vi "While Loop Stop Example.vi"() -> ()   [LabVIEW 2019]
uses:
  <vilib>/gpm_packages/@cs/test-executive/Source/Test Executive/TestExecutive/Test Executive.lvclass
  C:/Program Files/National Instruments/LabVIEW 2019/vi.lib/gpm_packages/@cs/test-executive/Source/Test Executive/ITestExecutive/ITest Executive.lvclass
  <vilib>/gpm_packages/@cs/run-time-assertions/Source/Assert Equal/Assert Equal.lvclass
  C:/Program Files/National Instruments/LabVIEW 2019/vi.lib/gpm_packages/@cs/run-time-assertions/Source/Assert/Assert.lvclass
  52cc7c55-fdef-40cb-9b01-06c8b27f6ce0.vi
  a0d94dfd-d8d0-4b1a-8204-38a80b6efbaa.vi
  c6de0239-6f38-4b7c-b092-4f7ec1379bf5.vi
  5f8b3cd8-e4ad-4ca2-853e-23f3d1aa975d.vi
  <vilib>/Utility/error.llb/Error Cluster From Error Code.vi
  <vilib>/gpm_packages/@cs/test-executive/Source/Test Executive/ITestExecutive/ITest Executive.lvclass
  <vilib>/gpm_packages/@cs/test-executive/Source/Test Executive/TestExecutive Ref/TestExecutive Ref.lvclass
  <vilib>/gpm_packages/@cs/test-executive/Source/Sandbox/While Loop Stop Example/Mock Executioner/Mock Executioner.lvclass
panel:
  in  "Stop":bool
  in  "Tree":string(tree)
  out "Iteration Counter":i32
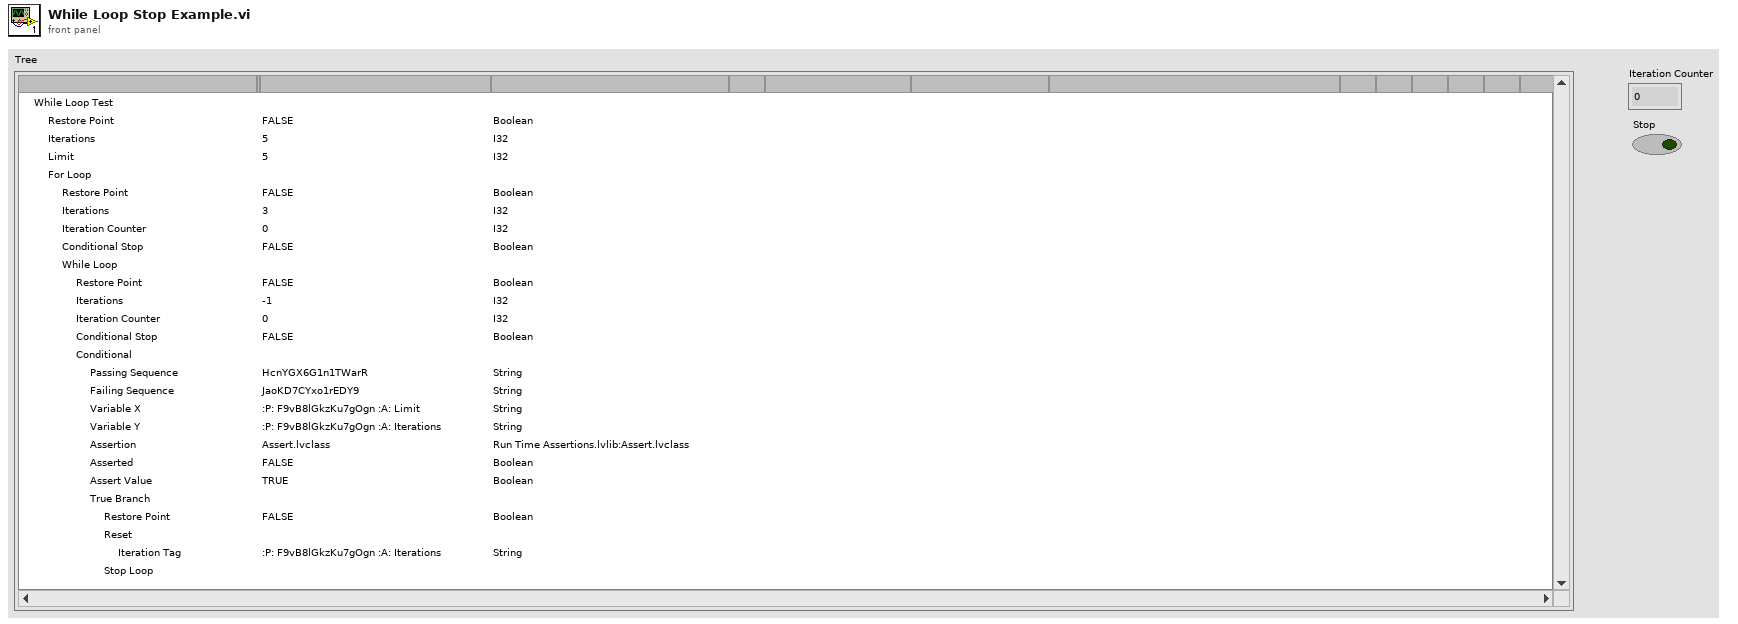
[diagram p1: front panel]
types:
  T1 = cluster{"Left Cell String":string, "Child Text":string[], "Child Tag":string, "Item Indent":i32, "Child Only?":bool, "Glyph Index":i32}[]
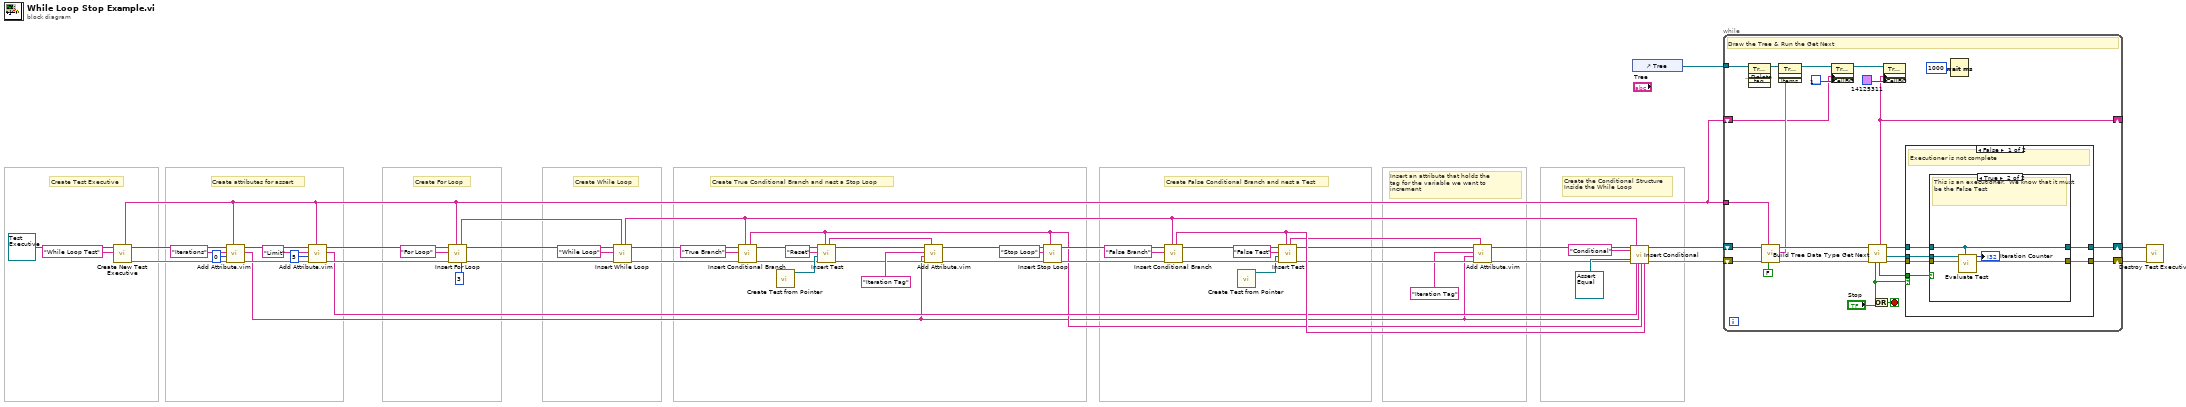
[diagram p0: block diagram]
diagram:
  # "Create For Loop"
  # "Insert an attribute that holds the\ntag for the variable we want to\nincrement"
  # "Create the Conditional Structure\nInside the While Loop"
  # "Create False Conditional Branch and nest a Test"
  # "Create True Conditional Branch and nest a Stop Loop"
  # "Create While Loop"
  # "Create attributes for assert"
  # "Create Test Executive"
  n1 = call <vilib>:"Create New Test Executive.vi"("Name"="While Loop Test", "Test Executive"=refnum<class "Test Executive.lvclass"> refnum ("Test Executive.lvlib:Test Executive.lvclass")) -> ("error out"=w54:errorcluster, "Test Executive Ref"=w55:refnum<data-value>, "Test Executive ID out"=w16:string)  [unwired: 7 in]
  n2 = call "Add Attribute.vim"("ID"=w16, "error in (no error)"=w54, "Attribute"=0, "Attribute Name"="Iterations", "Test Executive Ref"=w55) -> ("error out"=w45:errorcluster, "Attribute ID out"=w1:string, "Test Executive Ref out"=w46:refnum<data-value>)  [unwired: 3 in, 1 out]
  n3 = call "Add Attribute.vim"("ID"=w16, "error in (no error)"=w45, "Attribute"=5, "Attribute Name"="Limit", "Test Executive Ref"=w46) -> ("error out"=w22:errorcluster, "Attribute ID out"=w13:string, "Test Executive Ref out"=w20:refnum<data-value>)  [unwired: 3 in, 1 out]
  n4 = call <vilib>:"Insert For Loop.vi"("Loop Iterations"=3, "Parent ID"=w16, "error in (no error)"=w22, "Name"="For Loop", "Test Executive Ref"=w20) -> ("error out"=w21:errorcluster, "Test Executive Ref out"=w19:refnum<data-value>, "Unique ID out"=w15:string)  [unwired: 3 in, 1 out]
  n5 = call <vilib>:"Insert While Loop.vi"("Parent ID"=w15, "error in (no error)"=w21, "Name"="While Loop", "Test Executive Ref"=w19) -> ("error out"=w50:errorcluster, "Test Executive Ref out"=w51:refnum<data-value>, "Unique ID out"=w40:string)  [unwired: 4 in, 1 out]
  n6 = call <vilib>:"Insert Conditional Branch.vi"("Parent ID"=w40, "error in (no error)"=w50, "Name"="True Branch", "Test Executive Ref"=w51) -> ("error out"=w8:errorcluster, "Test Executive Ref out"=w10:refnum<data-value>, "Unique ID out"=w9:string)  [unwired: 4 in, 1 out]
  n7 = call <vilib>:"Create Test from Pointer.vi"() -> ("Test"=w12:refnum<class "Executioner.lvclass">)  [unwired: 11 in]
  n8 = call <vilib>:"Insert Test.vi"("Parent ID"=w9, "error in (no error)"=w8, "Test"=w12, "Name"="Reset", "Test Executive Ref"=w10) -> ("error out"=w4:errorcluster, "Test Executive Ref out"=w6:refnum<data-value>, "Unique ID out"=w2:string)  [unwired: 3 in, 1 out]
  n9 = call "Add Attribute.vim"("ID"=w2, "error in (no error)"=w4, "Attribute"=w1, "Attribute Name"="Iteration Tag", "Test Executive Ref"=w6) -> ("error out"=w3:errorcluster, "Test Executive Ref out"=w5:refnum<data-value>)  [unwired: 3 in, 2 out]
  n10 = call <vilib>:"Insert Stop Loop.vi"("Parent ID"=w9, "error in (no error)"=w3, "Name"="Stop Loop", "Test Executive Ref"=w5) -> ("error out"=w36:errorcluster, "Test Executive Ref out"=w14:refnum<data-value>)  [unwired: 4 in, 2 out]
  n11 = call <vilib>:"Insert Conditional Branch.vi"("Parent ID"=w40, "error in (no error)"=w36, "Name"="False Branch", "Test Executive Ref"=w14) -> ("error out"=w43:errorcluster, "Test Executive Ref out"=w42:refnum<data-value>, "Unique ID out"=w37:string)  [unwired: 4 in, 1 out]
  n12 = call <vilib>:"Create Test from Pointer.vi"() -> ("Test"=w29:refnum<class "Executioner.lvclass">)  [unwired: 11 in]
  n13 = call <vilib>:"Insert Test.vi"("Parent ID"=w37, "error in (no error)"=w43, "Test"=w29, "Name"="False Test", "Test Executive Ref"=w42) -> ("error out"=w32:errorcluster, "Test Executive Ref out"=w34:refnum<data-value>, "Unique ID out"=w30:string)  [unwired: 3 in, 1 out]
  n14 = call "Add Attribute.vim"("ID"=w30, "error in (no error)"=w32, "Attribute"=w1, "Attribute Name"="Iteration Tag", "Test Executive Ref"=w34) -> ("error out"=w31:errorcluster, "Test Executive Ref out"=w33:refnum<data-value>)  [unwired: 3 in, 2 out]
  n15 = call <vilib>:"Insert Conditional.vi"("Test Executive Ref"=w33, "Name"="Conditional", "Assertion"=refnum<class "Assert Equal.lvclass"> refnum ("Run Time Assertions.lvlib:Assert Equal.lvclass"), "error in (no error)"=w31, "Parent ID"=w40, "Variable X"=w13, "Variable Y"=w1, "Passing Executive"=w9, "Failing Executive"=w37) -> ("Test Executive Ref out"=w27:refnum<data-value>, "error out"=w26:errorcluster)  [unwired: 7 in, 2 out]
  n16 = control-ref of="Tree"() -> (w25:refnum<vi>)
  n17 = while {
    shift-right: [w78] -> w24
    shift-left: w27 -> [w76]
    shift-right: [w77] -> w23
    shift-left: w26 -> [w74]
    tunnel: w16 -> [w72]
    shift-right: [w62] -> _
    shift-left: w16 -> [w65]
    tunnel: w25 -> [w71]
    stop <- w61 stop-if-true
    # "Draw the Tree & Run the Get Next"
    n18 = invoke on="Invoke Node" class="Tree (strict)" method="Edit Tree Items.Delete"(reference=w71) -> (reference out=w70:refnum<vi>)  [unwired: 4 in, 4 out]
    n19 = call <vilib>:"Build Tree Data Type.vi"("Show IDs (True)"=FALSE, "Test ID"=w72, "error in (no error)"=w74, "Test Executive Ref"=w76) -> ("error out"=w73:errorcluster, "Tree Data"=w69:T1, "Test Executive Ref out"=w75:refnum<data-value>)  [unwired: 5 in]
    n20 = invoke on="Invoke Node" class="Tree (strict)" method="Edit Tree Items.Add Multiple Items to End"(reference=w70, "Items"=w69) -> (reference out=w66:refnum<vi>)  [unwired: 2 in, 3 out]
    n21 = property on="Property Node" class="Tree (strict)"(reference=w66, "Active Item Tag"=w65, "CellBG"=u32 16777226) -> (reference out=w63:refnum<vi>)  [unwired: 1 in, 1 out]
    n22 = call <vilib>:"Get Next.vi"("error in (no error)"=w73, "Test Executive Ref"=w75) -> ("error out"=w79:errorcluster, "Test"=w80:refnum<class "Executioner.lvclass">, "Test Executive Ref out"=w81:refnum<data-value>, "Found"=w82:bool, "Unique ID out"=w62:string, "Complete"=w83:bool)  [unwired: 3 in, 1 out]
    n23 = Or(x=w83, y="Stop") -> (x .or. y?=w61:bool)
    n24 = property on="Property Node" class="Tree (strict)"(reference=w63, "Active Item Tag"=w62, "CellBG"=u32 14125311) -> ()  [unwired: 1 in, 2 out]
    n25 = case shown="False" w83 {
      tunnel: w82 -> [w89 _]
      tunnel: w81 -> [w88 w97]
      tunnel: w80 -> [w87 _]
      tunnel: w79 -> [w86 w96]
      tunnel: [w85 w97] -> w78
      tunnel: [w84 w96] -> w77
      frame False {
        # "Executioner is not complete"
        n26 = case shown="True" w89 {
          tunnel: w88 -> [w91 w93]
          tunnel: w87 -> [_ w95]
          tunnel: w86 -> [w90 w92]
          tunnel: [w91 w93] -> w85
          tunnel: [w90 w92] -> w84
          frame False {
            # "This is not an executioner, ignore it"
          }
          frame True {
            # "This is an executioner.  We know that it must be the False Test"
            n27 = call <vilib>:"Evaluate Test.vi"("Test Executive Ref out"=w93, "Executioner in"=w95) -> ("Value"=→"Iteration Counter":i32)  [unwired: 9 in]
          }
        }
      }
      frame True {
        # "Executioner is complete, stop"
      }
    }
    n28 = Wait (ms)(milliseconds to wait=u32 1000) -> ()  [unwired: 1 out]
  }
  n29 = call <vilib>:"Destroy Test Executive.vi"("error in (no error)"=w23, "Test Executive Ref"=w24) -> ()  [unwired: 9 in, 1 out]
